vi "Configure Relative Reading.vi"(0 "VISA resource name":refnum<visa-resource-name>, 1 "Measurement (0: Voltage Channel 1)":i32(ring) items=["Voltage Channel 1", "Voltage Channel 2", "Temperature Channel 1", "Temperature Channel 2"], 5 "Enable Reference (F: Disable)":bool, 7 "Manually Set Reference (F: Disable)":bool, 9 "Reference Value (0)":dbl, 11 "error in (no error)":errorcluster) -> (4 "VISA resource name out":refnum<visa-resource-name>, 15 "error out":errorcluster)   [LabVIEW 2021, in "Keithley 2182.lvlib"]
doc: "Configures the measurement reference (Relative value) for the specified measurement.\n\nRelative (rel) nulls an offset or subtracts a baseline reading from present and future readings.\nWhen a rel value is established, subsequent readings will be the difference between the actual input and the rel value.\n\n<B>Displayed (Rel'ed) Reading = Actual Input - Rel Value</B>\n\nOnce a rel value is established for a measurement function, the value is the same for all ranges. For example, if 5V is set as the rel value on the 10V range for DCV1, the rel value is also 5V on the 100V, 1V, 100mV, and 10mV ranges.\n\nWhen a rel value is larger than the selected range, the display is formatted to accommodate the rel'd reading. However, this does not increase the maximum allowable input for that range.\nAn over-range input signal will still cause the display to overflow. For example, on the 10V range, the Model 2182 still overflows for a 12V input.\n\n<B>Note:</B>\nRel'ed readings are used for Ratio and Delta calculations."
uses:
  <instrlib>/Keithley 2182/Keithley 2182.lvlib
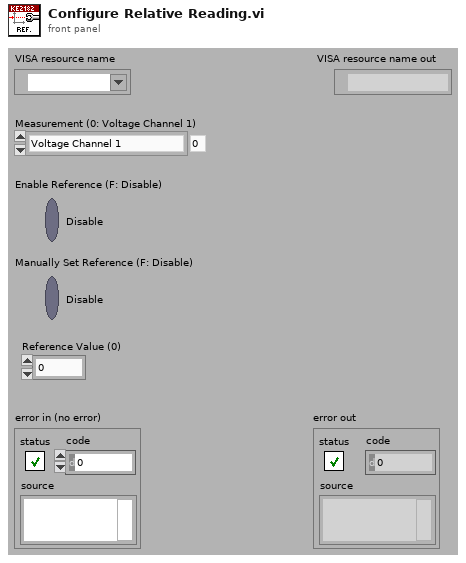
[diagram p1: front panel]
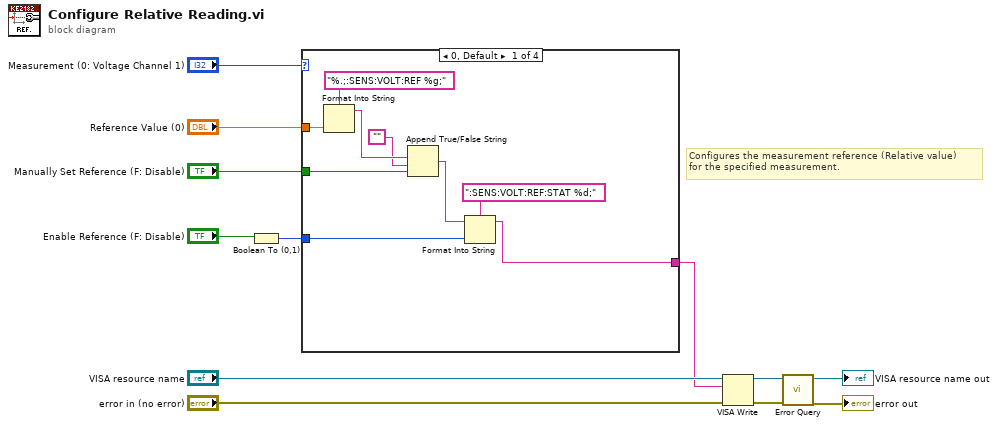
[diagram p0: block diagram]
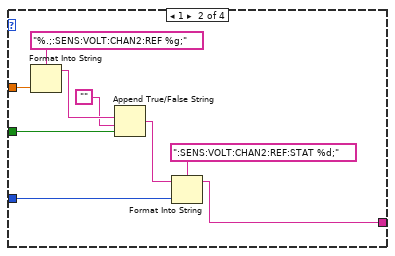
[diagram p2: hidden frame]
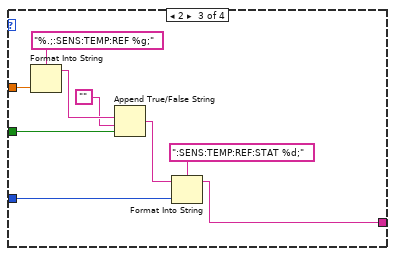
[diagram p3: hidden frame]
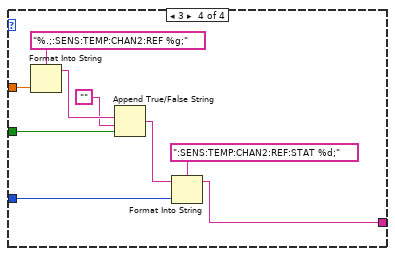
[diagram p4: hidden frame]
diagram:
  # "Configures the measurement reference (Relative value) \nfor the specified measurement."
  n1 = Boolean To (0,1)(Boolean="Enable Reference (F: Disable)") -> (0, 1=w4:i16)
  n2 = case shown="0, Default" "Measurement (0: Voltage Channel 1)" {
    tunnel: w4 -> [w21 w30 w39 w48]
    tunnel: "Reference Value (0)" -> [w19 w28 w37 w46]
    tunnel: [w13 w22 w31 w40] -> w2
    tunnel: "Manually Set Reference (F: Disable)" -> [w17 w26 w35 w44]
    frame 0, Default {
      n3 = Format Into String(format string="%.;:SENS:VOLT:REF %g;", w19) -> (resulting string=w16:string)  [unwired: 2 in, 1 out]
      n4 = Append True/False String(1:w17, 2:"", 3:w16) -> (0:w14:string)  [unwired: 1 in]
      n5 = Format Into String(format string=":SENS:VOLT:REF:STAT %d;", initial string=w14, w21) -> (resulting string=w13:string)  [unwired: 1 in, 1 out]
    }
    frame 1 {
      n6 = Format Into String(format string="%.;:SENS:VOLT:CHAN2:REF %g;", w28) -> (resulting string=w25:string)  [unwired: 2 in, 1 out]
      n7 = Append True/False String(1:w26, 2:"", 3:w25) -> (0:w23:string)  [unwired: 1 in]
      n8 = Format Into String(format string=":SENS:VOLT:CHAN2:REF:STAT %d;", initial string=w23, w30) -> (resulting string=w22:string)  [unwired: 1 in, 1 out]
    }
    frame 2 {
      n9 = Format Into String(format string="%.;:SENS:TEMP:REF %g;", w37) -> (resulting string=w34:string)  [unwired: 2 in, 1 out]
      n10 = Append True/False String(1:w35, 2:"", 3:w34) -> (0:w32:string)  [unwired: 1 in]
      n11 = Format Into String(format string=":SENS:TEMP:REF:STAT %d;", initial string=w32, w39) -> (resulting string=w31:string)  [unwired: 1 in, 1 out]
    }
    frame 3 {
      n12 = Format Into String(format string="%.;:SENS:TEMP:CHAN2:REF %g;", w46) -> (resulting string=w43:string)  [unwired: 2 in, 1 out]
      n13 = Append True/False String(1:w44, 2:"", 3:w43) -> (0:w41:string)  [unwired: 1 in]
      n14 = Format Into String(format string=":SENS:TEMP:CHAN2:REF:STAT %d;", initial string=w41, w48) -> (resulting string=w40:string)  [unwired: 1 in, 1 out]
    }
  }
  n15 = VISA Write(VISA resource name="VISA resource name", write buffer=w2, error in (no error)="error in (no error)") -> (VISA resource name out=w10:refnum<visa-resource-name>, error out=w9:errorcluster)  [unwired: 1 out]
  n16 = call <instrlib>:"Error Query.vi"("error in (no error)"=w9, "VISA resource name"=w10) -> ("error out"=→"error out":errorcluster, "VISA resource name out"=→"VISA resource name out":refnum<visa-resource-name>)  [unwired: 6 in, 2 out]
